vi "Lock-in query OVLD.vi"(8 "error in (no error)":errorcluster, 11 "Lockin SR830.lvclass In":refnum<class "Lockin SR830.lvclass">) -> (0 "error out":errorcluster, 2 "Ovld":bool=TRUE, 3 "Lockin SR830.lvclass out":refnum<class "Lockin SR830.lvclass">)   [LabVIEW 2017, in "SR830.lvlib"]
uses:
  Lockin SR830.lvclass
  SR830.lvlib
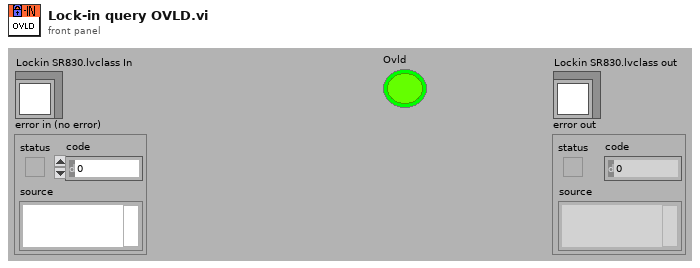
[diagram p1: front panel]
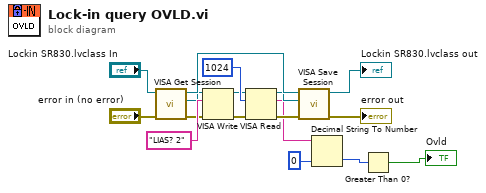
[diagram p0: block diagram]
diagram:
  n1 = call-dynamic "VISA Get Session.vi"("error in (no error)"="error in (no error)", "Instrument.lvclass in"="Lockin SR830.lvclass In") -> ("error out"=w9:errorcluster, "VISA Resource Name"=w10:refnum<visa-resource-name>, "Instrument.lvclass out"=w15:refnum<class "Lockin SR830.lvclass">)  [unwired: 6 in, 1 out]
  n2 = VISA Write(VISA resource name=w10, write buffer="LIAS? 2" ("data"), error in (no error)=w9) -> (VISA resource name out=w6:refnum<visa-resource-name>, error out=w7:errorcluster)  [unwired: 1 out]
  n3 = VISA Read(VISA resource name=w6, byte count=u32 1024, error in (no error)=w7) -> (VISA resource name out=w5:refnum<visa-resource-name>, read buffer=w3:string, error out=w4:errorcluster)  [unwired: 1 out]
  n4 = call-dynamic "VISA Save Session.vi"("error in (no error)"=w4, "VISA Resource Name"=w5, "Instrument.lvclass in"=w15) -> ("error out"=→"error out":errorcluster, "Instrument.lvclass out"=→"Lockin SR830.lvclass out":refnum<class "Lockin SR830.lvclass">)  [unwired: 7 in]
  n5 = Decimal String To Number(string=w3, default (0L)=u16 0 ("default (0 I32)")) -> (number=w2:u16)  [unwired: 1 in, 1 out]
  n6 = Greater Than 0?(x=w2) -> (x > 0?=→"Ovld":bool)
